vi "Analog Read Port.vi"(8 "Error In":errorcluster, 11 "ChipKit Resource":T1={"COM Port"="", "Board Type"=enum."ChipKit uC32", "Connection Type"=enum."USB / Serial", "Baud Rate (115200)"=15, "Bytes Per Packet (15)"=15}) -> (0 "Error Out":errorcluster, 2 "Analog Port":dbl[](array[numeric]), 3 "ChipKit Resource":T1={"COM Port"="", "Board Type"=enum."ChipKit uC32", "Connection Type"=enum."USB / Serial", "Baud Rate (115200)"=15, "Bytes Per Packet (15)"=15})   [LabVIEW 2011, in "LabVIEW Interface for ChipKit.lvlib"]
doc: "Read Arduino analog input port (A0 - A5)."
uses:
  LabVIEW Interface for ChipKit.lvlib
  Private/Type Defs/Command.ctl
  Private/Type Defs/Board Type.ctl
  Private/Type Defs/Chipkit Resource.ctl
  Private/Type Defs/Connection Type.ctl
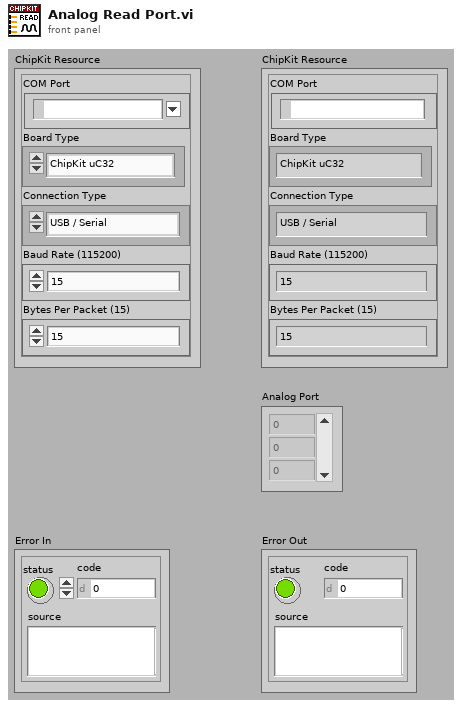
[diagram p1: front panel]
types:
  T1 = typedef "LabVIEW Interface for ChipKit.lvlib/Chipkit Resource.ctl" = cluster{"COM Port":refnum<visa-resource-name>, "Board Type":T2, "Connection Type":T3, "Baud Rate (115200)":u32, "Bytes Per Packet (15)":u32}
  T2 = typedef "LabVIEW Interface for ChipKit.lvlib/Board Type.ctl" = enum16{"ChipKit uC32", "ChipKit Uno32", "ChipKit Max32"}
  T3 = typedef "LabVIEW Interface for ChipKit.lvlib/Connection Type.ctl" = enum8{"USB / Serial", "XBEE", "BlueSmirf (Bluetooth)"}
  T4 = typedef "LabVIEW Interface for ChipKit.lvlib/Command.ctl" = enum8{"setArduinoMode", "flushSerial", "setPinMode", "digitalWritePin", "digitalWritePort", "tone", "digitalReadPin", "digitalReadPort", "analogReadPin", "analogReadPort", "pwmWritePin", "pwmWritePort", "sevenSegment_Configure", "sevenSegment_Write", "I2C Init", "I2C Write", "I2C Read", "SPI Init", "SPI Set Bit Order", "SPI Set Clock Divider", "SPI Set Data Mode", "SPI Send / Receive", "SPI Close", "Servo Set Num Servos", "Servo Config Servo", "Servo Write Angle", "Servo Read Angle", "Servo Write Pulse Width", "Servo Read Pulse Width", "Servo Detach", "LCD Init", "LCD Set Size", "LCD Set Cursor Mode", "LCD Clear", "LCD Set Cursor Position", "LCD Print", "LCD Display Power", "LCD Scroll Display", "LCD Autoscroll", "LCD Print Direction", "LCD Create Custom Char", "LCD Print Custom Char", "contAcqOn", "contAcqOff", "getFirmwareVersion", "FiniteSampleStart"}
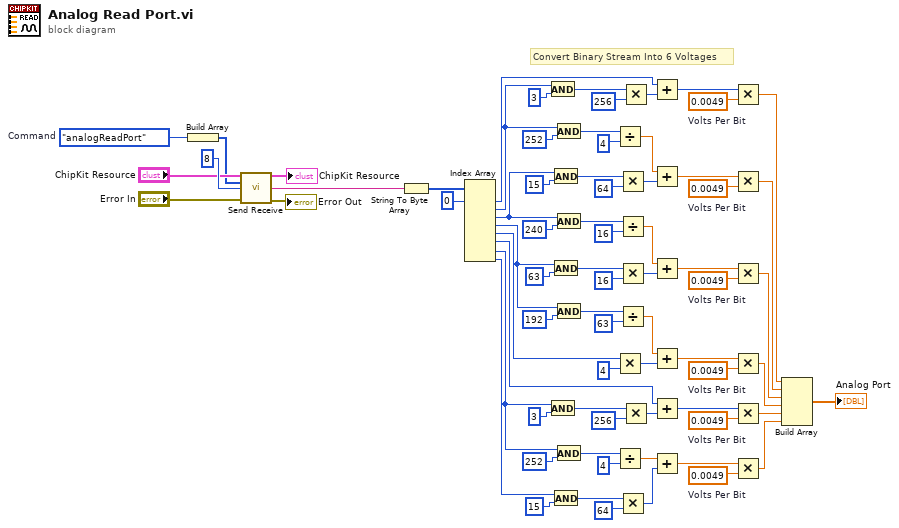
[diagram p0: block diagram]
diagram:
  w19 = 0.0049  # Volts Per Bit
  w31 = 0.0049  # Volts Per Bit
  w36 = 0.0049  # Volts Per Bit
  w52 = 0.0049  # Volts Per Bit
  w59 = 0.0049  # Volts Per Bit
  w70 = 0.0049  # Volts Per Bit
  w2 = Command."analogReadPort"  # Command
  # "Convert Binary Stream Into 6 Voltages"
  n1 = Build Array(w2) -> (w4:T4[])
  n2 = call "Send Receive.vi"("Arduino Resource"="ChipKit Resource", "Data"=w4, "Bytes To Read (0)"=u32 8, "error in"="Error In") -> ("Arduino Resource"=→"ChipKit Resource":T1, "Read Buffer"=w6:string, "error out"=→"Error Out":errorcluster)  [unwired: 9 in]
  n3 = String To Byte Array(string=w6) -> (unsigned byte array=w75:u8[])
  n4 = Index Array(array=w75, index #1=0 ("index")) -> (element #1=w68:u8, element #2=w66:u8, element #3=w55:u8, element #4=w33:u8, element #5=w24:u8, element #6=w23:u8, element #7=w12:u8, element #8=w11:u8)  [unwired: 7 in]
  n5 = And(x=w66, y=u8 3) -> (x .and. y?=w72:u8)
  n6 = And(x=w12, y=u8 3) -> (x .and. y?=w26:u8)
  n7 = And(x=w55, y=u8 15) -> (x .and. y?=w57:u8)
  n8 = And(x=w33, y=u8 63) -> (x .and. y?=w49:u8)
  n9 = And(x=w11, y=u8 15) -> (x .and. y?=w21:u8)
  n10 = And(x=w66, y=u8 252) -> (x .and. y?=w64:u8)
  n11 = And(x=w55, y=u8 240) -> (x .and. y?=w53:u8)
  n12 = And(x=w33, y=u8 192) -> (x .and. y?=w35:u8)
  n13 = And(x=w12, y=u8 252) -> (x .and. y?=w14:u8)
  n14 = Divide(x=w64, y=u8 4) -> (x/y=w56:dbl)
  n15 = Multiply(x=w24, y=u16 4) -> (x*y=w41:u16)
  n16 = Divide(x=w14, y=u8 4) -> (x/y=w22:dbl)
  n17 = Multiply(x=w57, y=u16 64) -> (x*y=w60:u16)
  n18 = Divide(x=w53, y=u8 16) -> (x/y=w50:dbl)
  n19 = Multiply(x=w49, y=u16 16) -> (x*y=w45:u16)
  n20 = Divide(x=w35, y=u8 63) -> (x/y=w38:dbl)
  n21 = Multiply(x=w21, y=u16 64) -> (x*y=w18:u16)
  n22 = Multiply(x=w72, y=u16 256) -> (x*y=w69:u16)
  n23 = Multiply(x=w26, y=u16 256) -> (x*y=w28:u16)
  n24 = Add(x=w68, y=w69) -> (x+y=w67:u16)
  n25 = Add(x=w56, y=w60) -> (x+y=w61:dbl)
  n26 = Add(x=w50, y=w45) -> (x+y=w51:dbl)
  n27 = Add(x=w38, y=w41) -> (x+y=w37:dbl)
  n28 = Add(x=w23, y=w28) -> (x+y=w30:u16)
  n29 = Add(x=w22, y=w18) -> (x+y=w17:dbl)
  n30 = Multiply(x=w67, y=w70) -> (x*y=w44:dbl)
  n31 = Multiply(x=w61, y=w59) -> (x*y=w43:dbl)
  n32 = Multiply(x=w51, y=w52) -> (x*y=w42:dbl)
  n33 = Multiply(x=w37, y=w36) -> (x*y=w32:dbl)
  n34 = Multiply(x=w30, y=w31) -> (x*y=w25:dbl)
  n35 = Multiply(x=w17, y=w19) -> (x*y=w10:dbl)
  n36 = Build Array(w44, w43, w42, w32, w25, w10) -> (→"Analog Port":dbl[])
